vi "Get Cells (1D Row String).vi"(8 "error in (no error)":errorcluster, 9 "Row":i32, 10 "Sheet Reference":refnum<k24>) -> (0 "error out":errorcluster, 2 "Sheet Reference out":refnum<k24>, 5 "Values":string[](array[string]))   [LabVIEW 2014]
uses:
  C:/PhaeronGit/LVNPOI/Resources/NPOI 2.1.1 dotnet2/NPOI.dll
  Resources/NPOI 2.1.1 dotnet2/NPOI.dll
  <vilib>/ErrorRing/Error Ring.xnode
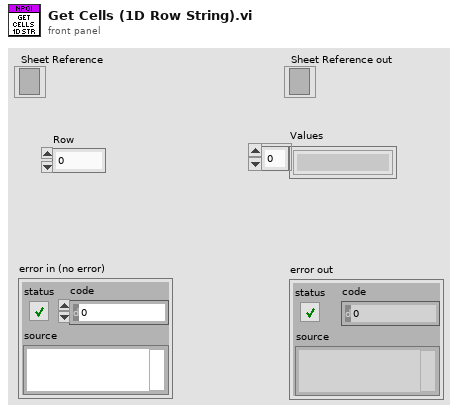
[diagram p1: front panel]
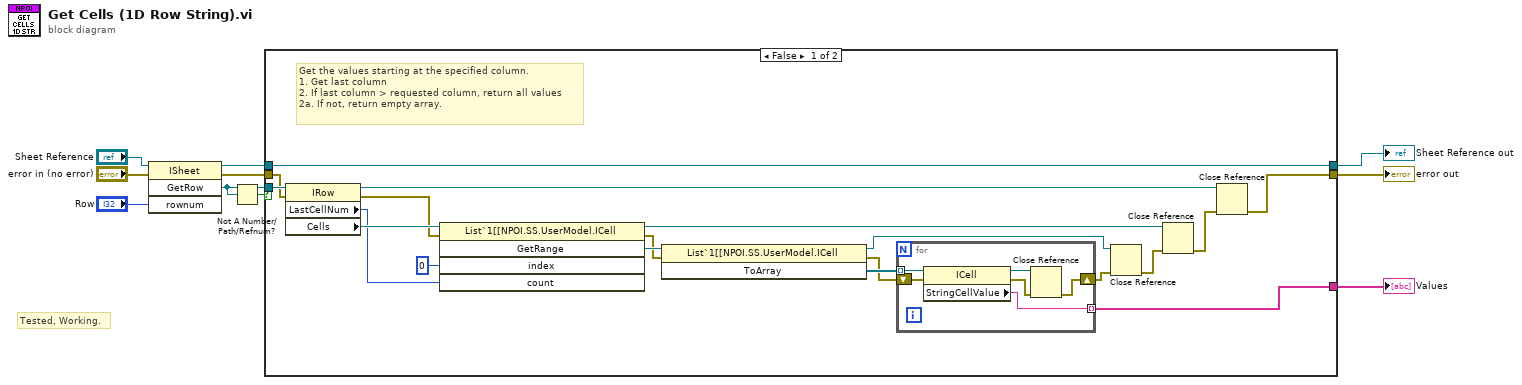
[diagram p0: block diagram]
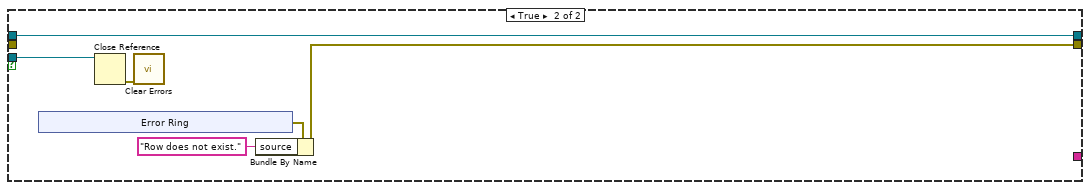
[diagram p2: hidden frame]
diagram:
  # "Tested, Working."
  n1 = invoke class="ISheet" method="GetRow"(reference="Sheet Reference", error in="error in (no error)", "rownum"="Row") -> (reference out=w7:refnum<k24>, error out=w8:errorcluster, "GetRow"=w10:refnum<k24>)  [unwired: 1 in, 1 out]
  n2 = Not A Number/Path/Refnum?(number/path/refnum=w10) -> (NaN/Path/Refnum?=w9:bool)
  n3 = case shown="False" w9 {
    tunnel: w7 -> [w22 w36]
    tunnel: w8 -> [w27 _]
    tunnel: [w23 w37] -> w1
    tunnel: [w22 w36] -> w3
    tunnel: w10 -> [w29 w38]
    tunnel: [w28 _] -> w2
    frame False {
      # "Get the values starting at the specified column.\n1. Get last column\n2. If last column > requested column, return all values\n2a. If not, return empty array."
      n4 = property class="IRow"(reference=w29, error in=w27) -> (reference out=w25:refnum<k24>, error out=w24:errorcluster, "LastCellNum"=w12:i16, "Cells"=w26:refnum<k24>)
      n5 = invoke class="List`1[[NPOI.SS.UserModel.ICell" method="GetRange"(reference=w26, error in=w24, "index"=0 ("Column"), "count"=w12) -> (reference out=w15:refnum<k24>, error out=w18:errorcluster, "GetRange"=w20:refnum<k24>)  [unwired: 1 in, 2 out]
      n6 = invoke class="List`1[[NPOI.SS.UserModel.ICell" method="ToArray"(reference=w20, error in=w18) -> (reference out=w17:refnum<k24>, error out=w19:errorcluster, "ToArray"=w21:refnum<k24>[])  [unwired: 1 in]
      n7 = for {
        tunnel: w21 -> [w35] mode=indexing
        tunnel: [w34] -> w28 mode=indexing
        shift-right: [w31] -> w16
        shift-left: w19 -> [w30]
        n8 = property class="ICell"(reference=w35, error in=w30) -> (reference out=w32:refnum<k24>, error out=w33:errorcluster, "StringCellValue"=w34:string)
        n9 = Close Reference(reference=w32, error in (no error)=w33) -> (error out=w31:errorcluster)
      }
      n10 = Close Reference(reference=w17, error in (no error)=w16) -> (error out=w14:errorcluster)
      n11 = Close Reference(reference=w15, error in (no error)=w14) -> (error out=w13:errorcluster)
      n12 = Close Reference(reference=w25, error in (no error)=w13) -> (error out=w23:errorcluster)
    }
    frame True {
      n13 = xnode "Error Ring"() -> ("error out"=w40:errorcluster)
      n14 = Close Reference(reference=w38) -> (error out=w39:errorcluster)  [unwired: 1 in]
      n15 = call <vilib>:"Clear Errors.vi"("error in (no error)"=w39) -> ()  [unwired: 5 in, 2 out]
      n16 = Bundle By Name(cluster=w40, "source"="Row does not exist.") -> (w37:errorcluster)
    }
  }
  "Sheet Reference out" <- w3
  "error out" <- w1
  "Values" <- w2
